vi "enumerateStaticDependencies.vi"(8 "error in (no error)":errorcluster, 11 "multichannel-lockin":refnum<class "multichannel-lockin.lvclass">) -> (0 "error out":errorcluster, 2 "Static Dependencies":refnum<class "Dependency.lvclass">[](array[class]), 3 "multichannel-lockin out":refnum<class "multichannel-lockin.lvclass">)   [LabVIEW 2019, in "multichannel-lockin.lvclass"]
doc: "JKI State Machine Objects (SMO) 1.3.0.56\nJKI - JKI\nCopyright (c) 2017, JKI"
uses:
  multichannel-lockin.lvclass
  <userlib>/LevyLab/Instrument Framework/SMOs/Instrument/Instrument.lvclass
  <vilib>/JKI/JKI SMO/Dependency/Dependency.lvclass
panel:
  # "For instructions on how to use the JKI State Machine Objects, examples and video tutorials, visit:\nhttp://jki.net/state-machine-objects/\n\nJKI State Machine Objects™\nhttp://jki.net/state-machine-objects/\nCopyright (C) 2005-2015, JKI <info@jki.net>\nALL RIGHTS RESERVED"
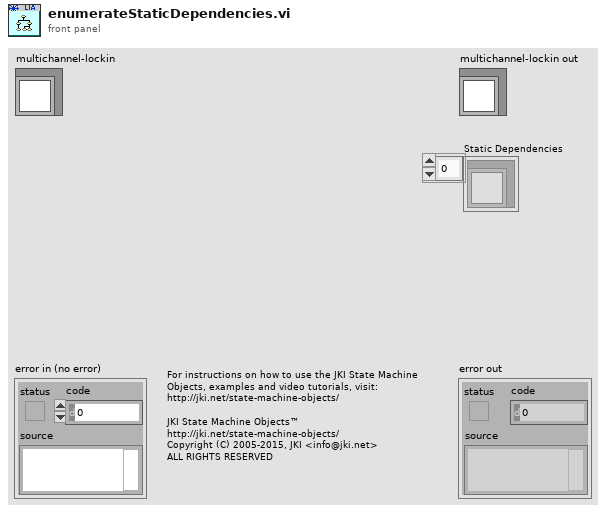
[diagram p1: front panel]
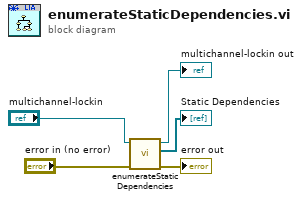
[diagram p0: block diagram]
diagram:
  n1 = call-parent "enumerateStaticDependencies.vi"("error in (no error)"="error in (no error)", "Instrument"="multichannel-lockin") -> ("error out"=→"error out":errorcluster, "Static Dependencies"=→"Static Dependencies":refnum<class "Dependency.lvclass">[], "Instrument out"=→"multichannel-lockin out":refnum<class "multichannel-lockin.lvclass">)  [unwired: 7 in]
